vi "Begin.vi"(11 "Image Size":T1=enum."160x120") -> (0 "error out":errorcluster)   [LabVIEW 2012]
doc: "Called before other user functions, this VI is expected to open initial I/O refnums, load in file data, and do all program initialization. Notice that the <B>error out</B> terminal is simply used for data flow. Wiring it to other structures or subVIs ensures that this VI runs first."
uses:
  <vilib>/Rock Robotics/WPI/Camera/WPI_CameraImageSize.ctl
  <vilib>/Rock Robotics/WPI/Camera/WPI_CameraWhite Balance Values.ctl
  <vilib>/Rock Robotics/WPI/Camera/WPI_CameraExposure Values.ctl
  <vilib>/Rock Robotics/WPI/Camera/WPI_CameraFrameRate.ctl
  <vilib>/Rock Robotics/WPI/DriverStation/WPI_DriverStationRobotMode2.ctl
  <vilib>/Rock Robotics/WPI/Joystick/WPI_JoystickDeviceEnum.ctl
  <vilib>/Rock Robotics/SystemInterfaces/Typedef/FPGA_TypedefDigitalModule.ctl
  <vilib>/Rock Robotics/SystemInterfaces/DIO/FPGA_DIOPWMChannel.ctl
  <vilib>/Rock Robotics/WPI/Solenoid/WPI_SolenoidChannel.ctl
  <vilib>/Rock Robotics/SystemInterfaces/Typedef/FPGA_TypedefSolenoidModule.ctl
  <vilib>/Rock Robotics/SystemInterfaces/DIO/FPGA_DIOChannel.ctl
  <vilib>/Rock Robotics/WPI/Encoder/WPI_EncoderType.ctl
  <vilib>/Rock Robotics/WPI/SafetyOutput/WPI_SafetyOutputConfigMenu.ctl
  <vilib>/Rock Robotics/WPI/Solenoid/WPI_SolenoidValue.ctl
  <vilib>/Rock Robotics/SystemInterfaces/DIO/FPGA_DIORelayChannel.ctl
  <vilib>/Rock Robotics/SystemInterfaces/Typedef/FPGA_TypedefAnalogModuleForGyro.ctl
  <vilib>/Rock Robotics/SystemInterfaces/AI/FPGA_AIGyroChannel.ctl
  Robot Global Data.vi
  <vilib>/Rock Robotics/WPI/Solenoid/WPI_SolenoidOpenSingle.vi
  <vilib>/Rock Robotics/WPI/Solenoid/WPI_SolenoidSetEnum.vi
  <vilib>/Rock Robotics/WPI/Counter/WPI_CounterDigitalInputToDigitalSource.vi
  <vilib>/Rock Robotics/WPI/RobotDrive/WPI_RobotDriveOpen2MotorWithTalon.vi
  <vilib>/Rock Robotics/WPI/Solenoid/WPI_SolenoidOpenDouble.vi
  <vilib>/Rock Robotics/WPI/MotorControl/WPI_MotorControlOpen Talon.vi
  <vilib>/Rock Robotics/WPI/Compressor/WPI_CompressorGetSetRefNum.vi
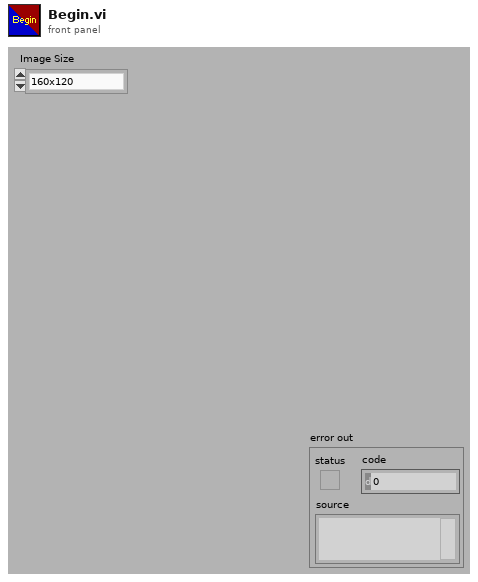
[diagram p1: front panel]
types:
  T1 = typedef "WPI_CameraImageSize.ctl" = enum16{"640x480", "320x240", "160x120"}
  T2 = typedef "WPI_SolenoidChannel.ctl" = enum8{"Solenoid 1", "Solenoid 2", "Solenoid 3", "Solenoid 4", "Solenoid 5", "Solenoid 6", "Solenoid 7", "Solenoid 8", "Invalid"}
  T3 = typedef "WPI_SolenoidValue.ctl" = enum16{"Off", "On", "Forward", "Reverse"}
  T4 = typedef "FPGA_AIGyroChannel.ctl" = enum8{"AI 1", "AI 2", "Invalid"}
  T5 = typedef "FPGA_TypedefAnalogModuleForGyro.ctl" = enum16{"Analog Module 1"}
  T6 = typedef "FPGA_DIOChannel.ctl" = enum8{"DIO 1", "DIO 2", "DIO 3", "DIO 4", "DIO 5", "DIO 6", "DIO 7", "DIO 8", "DIO 9", "DIO 10", "DIO 11", "DIO 12", "DIO 13", "DIO 14", "Invalid"}
  T7 = typedef "FPGA_DIORelayChannel.ctl" = enum8{"Relay 1", "Relay 2", "Relay 3", "Relay 4", "Relay 5", "Relay 6", "Relay 7", "Relay 8", "Invalid"}
  T8 = typedef "FPGA_TypedefDigitalModule.ctl" = enum16{"Digital Module 1", "Digital Module 2"}
  T9 = typedef "WPI_SafetyOutputConfigMenu.ctl" = enum16{"Enable", "Disable"}
  T10 = typedef "FPGA_DIOPWMChannel.ctl" = enum8{"PWM 1", "PWM 2", "PWM 3", "PWM 4", "PWM 5", "PWM 6", "PWM 7", "PWM 8", "PWM 9", "PWM 10", "Invalid"}
  T11 = typedef "WPI_EncoderType.ctl" = enum16{"1x", "2x", "4x"}
  T12 = typedef "FPGA_TypedefSolenoidModule.ctl" = enum16{"Solenoid Module 1", "Solenoid Module 2"}
  T13 = typedef "WPI_JoystickDeviceEnum.ctl" = enum16{"USB 1", "USB 2", "USB 3", "USB 4", "Kinect 1", "Kinect 2"}
  T14 = typedef "WPI_DriverStationRobotMode2.ctl" = enum16{"Autonomous Disabled", "Autonomous Enabled", "Teleop Disabled", "Teleop Enabled", "Timeout", "Finish", "Test Disabled", "Test Enabled"}
  T15 = typedef "WPI_CameraFrameRate.ctl" = u32
  T16 = typedef "WPI_CameraExposure Values.ctl" = enum16{"Auto", "Flicker-free 50 Hz", "Flicker-free 60 Hz", "Hold current"}
  T17 = typedef "WPI_CameraWhite Balance Values.ctl" = enum16{"Auto", "Fixed indoor", "Fixed outdoor 1", "Fixed outdoor 2", "Fixed fluorescent 1", "Fixed fluorescent 2", "Hold current"}
  T18 = typedef "WPI_DigitalInputDevRef.ctl" = cluster{"DevStatus":errorcluster, "DIO Channel":T6, "Digital Module":T8}
  T19 = typedef "WPI_CompressorDevRef.ctl" = cluster{"DevStatus":errorcluster, "DigitalInputDevRef":T18, "RelayDevRef":T20}
  T20 = typedef "WPI_RelayDevRef.ctl" = cluster{"DevStatus":errorcluster, "Relay Channel":T7, "Digital Module":T8, "Relay Direction":T21}
  T21 = typedef "WPI_RelayDirection.ctl" = enum16{"Both directions", "Forward only", "Reverse only"}
  T22 = typedef "FPGA_CounterEncoderSourceConvertionLVSourceType.ctl" = cluster{"DevStatus":errorcluster, "AnalogTriggerMode?":bool, "DigitalMode":cluster{"Digital Module":T8, "DIO Channel":T23}, "AnalogTriggerMode":cluster{"AnalogTriggerIndex":T24, "OutputType":T25}}
  T23 = typedef "FPGA_DIODigitalSourceChannel.ctl" = enum8{"DIO 1", "DIO 2", "DIO 3", "DIO 4", "DIO 5", "DIO 6", "DIO 7", "DIO 8", "DIO 9", "DIO 10", "DIO 11", "DIO 12", "DIO 13", "DIO 14", "Disabled"}
  T24 = typedef "FPGA_AnalogTriggerIndex.ctl" = enum8{"Trig 0", "Trig 1", "Trig 2", "Trig 3", "Trig 4", "Trig 5", "Trig 6", "Trig 7", "Invalid"}
  T25 = typedef "FPGA_AnalogTriggerOutType.ctl" = enum16{"InWindow", "TriggerState", "Rising", "Falling"}
  T26 = typedef "WPI_JoystickDevRef.ctl" = cluster{"Device":T13}
  T27 = typedef "WPI_CameraDevRef.ctl" = cluster{"Camera Address":string, "CameraStatus":errorcluster, "Acquire Image Notifier":refnum<notifier>}
  T28 = typedef "WPI_RobotDriveDevRef.ctl" = cluster{"DevStatus":errorcluster, "Motors[]":T29[], "Square Inputs":bool, "Max Output":dbl, "Isochronous":bool}
  T29 = typedef "WPI_MotorControlDeviceRef.ctl" = cluster{"DeviceStatus":errorcluster, "Type":enum16{"PWM", "CAN"}, "PWM":cluster{"Digital Module":T8, "PWM Channel":T10, "DeadBand":T30}, "CAN":cluster{"Device Number":u8, "Control Mode":T31, "Semaphore":T32, "Max Vout":dbl}, "Invert":bool, "TransformRef":T33, "InvTransformRef":T33}
  T30 = typedef "WPI_PWMDeadband.ctl" = cluster{"Name":string, "maxPositivePwm":i32, "minPositivePwm":i32, "centerPwm":i32, "maxNegativePwm":i32, "minNegativePwm":i32, "angularRange":u16}
  T31 = typedef "WPI_CANJaguar_ControlMode.ctl" = enum8{"Percent VBus", "Current", "Speed", "Position", "Voltage"}
  T32 = typedef "Semaphore RefNum" = refnum<k1>
  T33 = typedef "WPI_PWMTransform_ConPane.ctl" = refnum<vi>
  T34 = typedef "WPI_EncoderDevRef.ctl" = cluster{"DevStatus":errorcluster, "EncoderIndex":T35, "CounterIndex":T36, "DistancePerCount":dbl, "Decoding Type":T11}
  T35 = typedef "FPGA_EncoderIdx.ctl" = enum8{"Enc 0", "Enc 1", "Enc 2", "Enc 3", "Invalid"}
  T36 = typedef "FPGA_CounterCtrSystemIndex.ctl" = enum8{"Ctr 0", "Ctr 1", "Ctr 2", "Ctr 3", "Ctr 4", "Ctr 5", "Ctr 6", "Ctr 7", "Invalid"}
  T37 = typedef "WPI_SolenoidDevRef.ctl" = cluster{"DevStatus":errorcluster, "Solenoid Module":T12, "Forward Solenoid Channel":T2, "Reverse Solenoid Channel":T2}
  T38 = typedef "WPI_GyroDevRef.ctl" = cluster{"DevStatus":errorcluster, "Analog Module":T39, "Analog Channel":T40, "Offset":dbl, "Gain (VoltsPerDegree/Second)":dbl}
  T39 = typedef "FPGA_TypedefAnalogModule.ctl" = enum16{"Analog Module 1", "Analog Module 2"}
  T40 = typedef "FPGA_AIChannel.ctl" = enum8{"AI 1", "AI 2", "AI 3", "AI 4", "AI 5", "AI 6", "AI 7", "AI 8", "Invalid"}
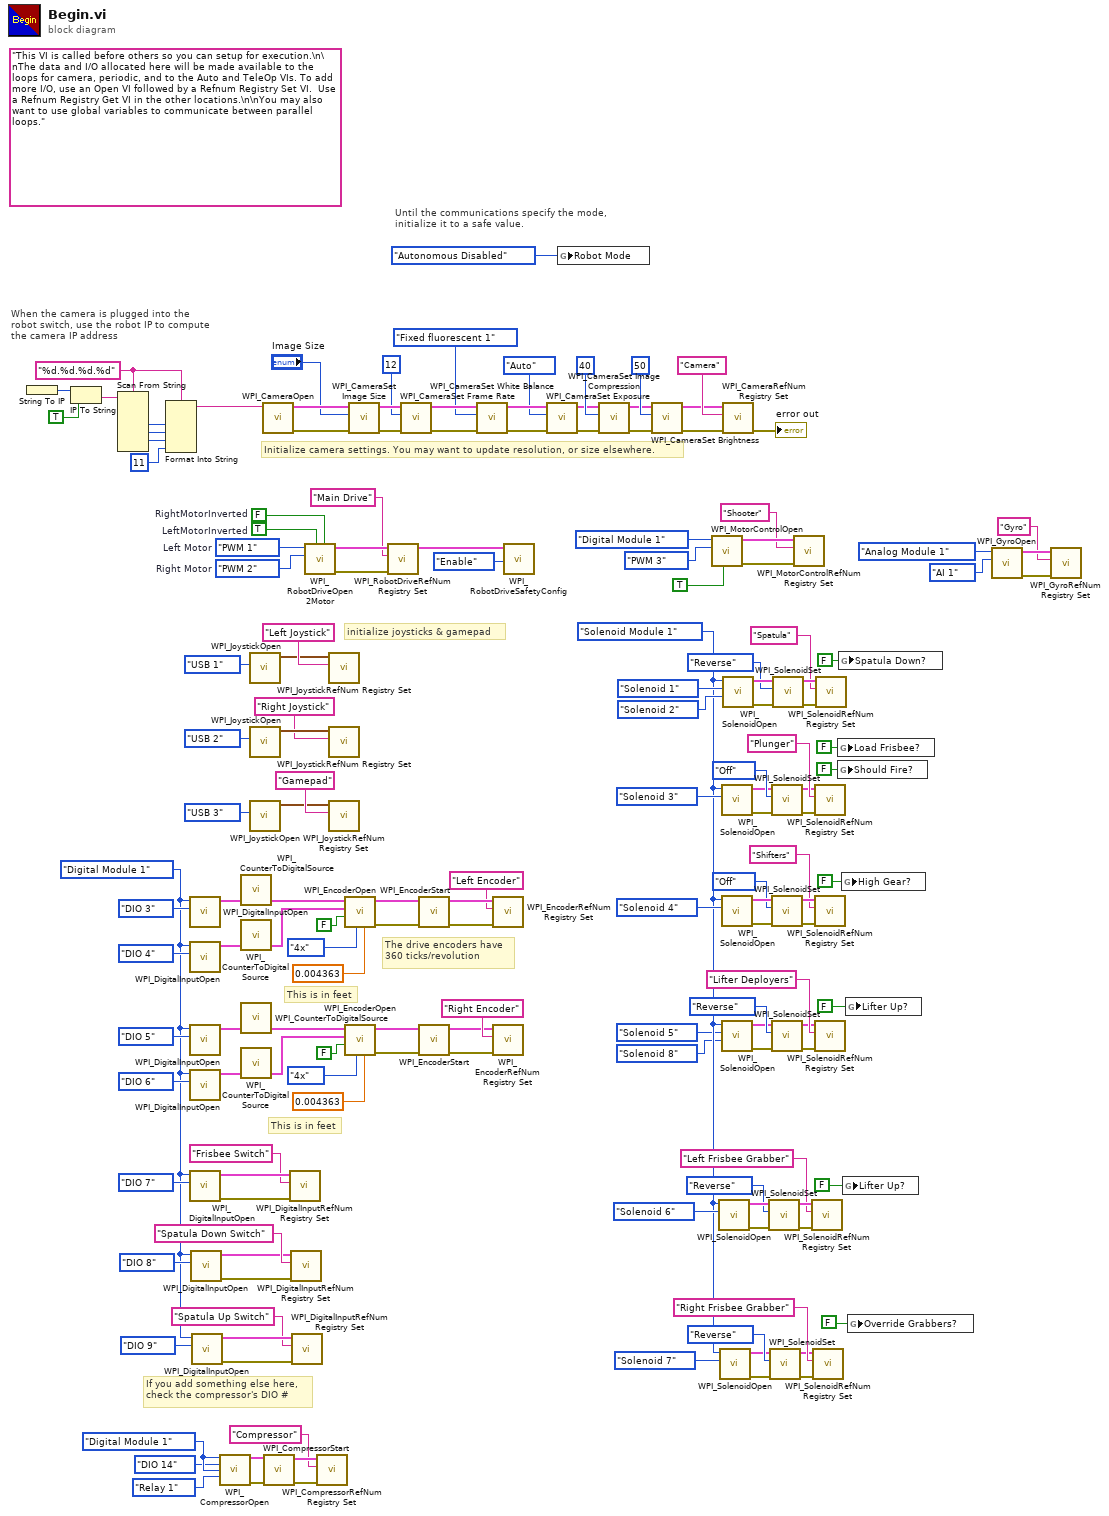
[diagram p0: block diagram]
diagram:
  w49 = FPGA_TypedefDigitalModule."Digital Module 1" ("Pressure Switch Digital Module (Module 1)")
  w67 = FPGA_DIOPWMChannel."PWM 2"  # Right Motor
  w68 = FPGA_DIOPWMChannel."PWM 1"  # Left Motor
  w72 = TRUE  # LeftMotorInverted
  w73 = FALSE  # RightMotorInverted
  w10 = FPGA_TypedefSolenoidModule."Solenoid Module 1" ("Solenoid Module (Module 1)")
  w33 = FPGA_TypedefDigitalModule."Digital Module 1" ("Digital Module (Module 1)")
  w134 = "%d.%d.%d.%d" ("format string")
  (unwired) "This VI is called before others so you can setup for execution.\n\nThe data and I/O allocated here will be made available to the loops for camera, periodic, and to the Auto and TeleOp VIs. To add more I/O, use an Open VI followed by a Refnum Registry Set VI.  Use a Refnum Registry Get VI in the other locations.\n\nYou may also want to use global variables to communicate between parallel loops."
  # "If you add something else here,\ncheck the compressor's DIO #"
  # "The drive encoders have\n360 ticks/revolution"
  # "This is in feet"
  # "This is in feet"
  # "initialize joysticks & gamepad"
  # "Until the communications specify the mode,\ninitialize it to a safe value."
  # "When the camera is plugged into the\nrobot switch, use the robot IP to compute\nthe camera IP address"
  # "Initialize camera settings. You may want to update resolution, or size elsewhere."
  n1 = String To IP() -> (0:w141:u32)  [unwired: 1 in]
  n2 = IP To String(1:TRUE ("dot notation? (F)"), 2:w141) -> (0:w139:string)
  n3 = Scan From String(format string=w134, input string=w139) -> (output 1=w138:i32, output 2=w137:i32, output 3=w136:i32)  [unwired: 7 in, 3 out]
  n4 = Format Into String(format string=w134, w138, w137, w136, 11 ("Compression")) -> (resulting string=w132:string)  [unwired: 2 in, 1 out]
  n5 = call <vilib>:"WPI_DigitalInputOpen.vi"("DIO Channel"=FPGA_DIOChannel."DIO 3" ("CS Channel"), "Digital Module (Module 1)"=w33) -> ("DigitalInputDevRef"=w95:T18)  [unwired: 1 in, 8 out]
  n6 = call <vilib>:"WPI_DigitalInputOpen.vi"("DIO Channel"=FPGA_DIOChannel."DIO 4" ("Clock Channel"), "Digital Module (Module 1)"=w33) -> ("DigitalInputDevRef"=w96:T18)  [unwired: 1 in, 8 out]
  n7 = call <vilib>:"WPI_DigitalInputOpen.vi"("DIO Channel"=FPGA_DIOChannel."DIO 5" ("CS Channel"), "Digital Module (Module 1)"=w33) -> ("DigitalInputDevRef"=w80:T18)  [unwired: 1 in, 8 out]
  n8 = call <vilib>:"WPI_DigitalInputOpen.vi"("DIO Channel"=FPGA_DIOChannel."DIO 6" ("Clock Channel"), "Digital Module (Module 1)"=w33) -> ("DigitalInputDevRef"=w79:T18)  [unwired: 1 in, 8 out]
  n9 = call <vilib>:"WPI_DigitalInputOpen.vi"("DIO Channel"=FPGA_DIOChannel."DIO 7", "Digital Module (Module 1)"=w33) -> ("error out"=w51:errorcluster, "DigitalInputDevRef"=w52:T18)  [unwired: 8 in]
  n10 = call <vilib>:"WPI_DigitalInputOpen.vi"("DIO Channel"=FPGA_DIOChannel."DIO 8", "Digital Module (Module 1)"=w33) -> ("error out"=w40:errorcluster, "DigitalInputDevRef"=w39:T18)  [unwired: 8 in]
  n11 = call <vilib>:"WPI_DigitalInputOpen.vi"("DIO Channel"=FPGA_DIOChannel."DIO 9", "Digital Module (Module 1)"=w33) -> ("error out"=w35:errorcluster, "DigitalInputDevRef"=w36:T18)  [unwired: 8 in]
  n12 = call <vilib>:"WPI_CompressorOpen.vi"("Pressure Switch Digital Module (Module 1)"=w49, "Pressure Switch DIO Channel"=FPGA_DIOChannel."DIO 14", "Relay Digital Module (Module 1)"=w49, "Relay Channel"=FPGA_DIORelayChannel."Relay 1") -> ("CompressorDevRef"=w45:T19, "error out"=w46:errorcluster)  [unwired: 10 in]
  n13 = call-poly <vilib>:"WPI_CounterToDigitalSource.vi"("DigitalInputDevRef"=w95) -> ("Digital Source"=w92:T22)  [unwired: 6 out]
  n14 = call-poly <vilib>:"WPI_CounterToDigitalSource.vi"("DigitalInputDevRef"=w96) -> ("Digital Source"=w93:T22)  [unwired: 6 out]
  n15 = call-poly <vilib>:"WPI_CounterToDigitalSource.vi"("DigitalInputDevRef"=w80) -> ("Digital Source"=w83:T22)  [unwired: 6 out]
  n16 = call-poly <vilib>:"WPI_CounterToDigitalSource.vi"("DigitalInputDevRef"=w79) -> ("Digital Source"=w82:T22)  [unwired: 6 out]
  n17 = call <vilib>:"WPI_JoystickOpen.vi"("JoystickDevice"=WPI_JoystickDeviceEnum."USB 1") -> ("JoystickDevRef"=w130:T26)  [unwired: 10 in]
  n18 = call <vilib>:"WPI_JoystickOpen.vi"("JoystickDevice"=WPI_JoystickDeviceEnum."USB 2") -> ("JoystickDevRef"=w126:T26)  [unwired: 10 in]
  n19 = call <vilib>:"WPI_JoystickOpen.vi"("JoystickDevice"=WPI_JoystickDeviceEnum."USB 3") -> ("JoystickDevRef"=w123:T26)  [unwired: 10 in]
  n20 = call <vilib>:"WPI_CameraOpen.vi"("Camera Address"=w132) -> ("error out"=w153:errorcluster, "CameraDevRef"=w154:T27)  [unwired: 1 in, 8 out]
  n21 = call <vilib>:"WPI_CompressorStart.vi"("error in (no error)"=w46, "CompressorDevRef"=w45) -> ("error out"=w44:errorcluster, "CompressorDevRef"=w43:T19)  [unwired: 8 in]
  n22 = call <vilib>:"WPI_DigitalInputRefNum Registry Set.vi"("error in (no error)"=w51, "refnum name"="Frisbee Switch", "DigitalInputDevRef"=w52) -> ()  [unwired: 7 in, 2 out]
  n23 = call <vilib>:"WPI_DigitalInputRefNum Registry Set.vi"("error in (no error)"=w40, "refnum name"="Spatula Down Switch", "DigitalInputDevRef"=w39) -> ()  [unwired: 7 in, 2 out]
  n24 = call <vilib>:"WPI_DigitalInputRefNum Registry Set.vi"("error in (no error)"=w35, "refnum name"="Spatula Up Switch", "DigitalInputDevRef"=w36) -> ()  [unwired: 7 in, 2 out]
  n25 = call-poly <vilib>:"WPI_RobotDriveOpen2Motor.vi"("Right Motor Inverted"=w73, "Left Motor Inverted"=w72, "Right Motor"=w67, "Left Motor"=w68) -> ("error out"=w69:errorcluster, "RobotDriveDevRef"=w71:T28)  [unwired: 1 in, 5 out]
  n26 = call <vilib>:"WPI_CompressorRefNum Registry Set.vi"("error in (no error)"=w44, "refnum name"="Compressor", "CompressorDevRef"=w43) -> ()  [unwired: 7 in, 2 out]
  n27 = call <vilib>:"WPI_JoystickRefNum Registry Set.vi"("refnum name"="Left Joystick", "JoystickDevRef"=w130) -> ()  [unwired: 8 in, 2 out]
  n28 = call <vilib>:"WPI_JoystickRefNum Registry Set.vi"("refnum name"="Right Joystick", "JoystickDevRef"=w126) -> ()  [unwired: 8 in, 2 out]
  n29 = call <vilib>:"WPI_JoystickRefNum Registry Set.vi"("refnum name"="Gamepad", "JoystickDevRef"=w123) -> ()  [unwired: 8 in, 2 out]
  n30 = call <vilib>:"WPI_EncoderOpen.vi"("DistancePerCount"=0.004363, "Decoding Type"=WPI_EncoderType."4x", "Invert Direction (False)"=FALSE, "BSource"=w93, "ASource"=w92) -> ("error out"=w98:errorcluster, "EncoderDevRef"=w97:T34)  [unwired: 5 in]
  n31 = call <vilib>:"WPI_EncoderOpen.vi"("DistancePerCount"=0.004363, "Decoding Type"=WPI_EncoderType."4x", "Invert Direction (False)"=FALSE, "BSource"=w82, "ASource"=w83) -> ("error out"=w77:errorcluster, "EncoderDevRef"=w78:T34)  [unwired: 5 in]
  n32 = call <vilib>:"WPI_CameraSet Image Size.vi"("error in (no error)"=w153, "Image Size"="Image Size", "CameraDevRef"=w154) -> ("error out"=w152:errorcluster, "CameraDevRef Out"=w155:T27)  [unwired: 7 out]
  n33 = call <vilib>:"WPI_RobotDriveRefNum Registry Set.vi"("error in (no error)"=w69, "refnum name"="Main Drive", "RobotDriveDevRef"=w71) -> ("RobotDriveDevRef"=w66:T28)  [unwired: 8 out]
  n34 = call <vilib>:"WPI_CameraSet Frame Rate.vi"("error in (no error)"=w152, "Frame Rate (fps)"=T15 12, "CameraDevRef"=w155) -> ("error out"=w151:errorcluster, "CameraDevRef Out"=w157:T27)  [unwired: 7 out]
  n35 = call <vilib>:"WPI_EncoderStart.vi"("error in (no error)"=w98, "EncoderDevRef"=w97) -> ("error out"=w99:errorcluster, "EncoderDevRef"=w100:T34)  [unwired: 8 in]
  n36 = call <vilib>:"WPI_EncoderStart.vi"("error in (no error)"=w77, "EncoderDevRef"=w78) -> ("error out"=w76:errorcluster, "EncoderDevRef"=w75:T34)  [unwired: 8 in]
  n37 = call <vilib>:"WPI_CameraSet White Balance.vi"("error in (no error)"=w151, "White Balance"=WPI_CameraWhite_Balance_Values."Fixed fluorescent 1", "CameraDevRef"=w157) -> ("error out"=w150:errorcluster, "CameraDevRef Out"=w156:T27)  [unwired: 7 out]
  n38 = call <vilib>:"WPI_EncoderRefNum Registry Set.vi"("error in (no error)"=w99, "refnum name"="Left Encoder", "EncoderDevRef"=w100) -> ()  [unwired: 7 in, 2 out]
  n39 = call <vilib>:"WPI_EncoderRefNum Registry Set.vi"("error in (no error)"=w76, "refnum name"="Right Encoder", "EncoderDevRef"=w75) -> ()  [unwired: 7 in, 2 out]
  n40 = call <vilib>:"WPI_RobotDriveSafetyConfig.vi"("mode"=WPI_SafetyOutputConfigMenu."Enable", "RobotDriveDevRef"=w66) -> ()  [unwired: 8 in, 2 out]
  n41 = call <vilib>:"WPI_CameraSet Exposure.vi"("error in (no error)"=w150, "Exposure"=WPI_CameraExposure_Values."Auto", "CameraDevRef"=w156) -> ("error out"=w149:errorcluster, "CameraDevRef Out"=w159:T27)  [unwired: 7 out]
  n42 = global write "Robot Global Data.vi" "Robot Mode"(WPI_DriverStationRobotMode2."Autonomous Disabled" ("Robot Mode")) -> ()
  n43 = call <vilib>:"WPI_CameraSet Image Compression.vi"("error in (no error)"=w149, "Compression"=40, "CameraDevRef"=w159) -> ("error out"=w148:errorcluster, "CameraDevRef Out"=w158:T27)  [unwired: 7 out]
  n44 = call <vilib>:"WPI_CameraSet Brightness.vi"("error in (no error)"=w148, "Brightness"=50, "CameraDevRef"=w158) -> ("error out"=w146:errorcluster, "CameraDevRef Out"=w147:T27)  [unwired: 7 out]
  n45 = call-poly <vilib>:"WPI_MotorControlOpen.vi"("Invert"=TRUE, "PWM Channel"=FPGA_DIOPWMChannel."PWM 3", "Digital Module (Module 1)"=FPGA_TypedefDigitalModule."Digital Module 1") -> ("error out"=w118:errorcluster, "MotorControlDeviceRef"=w119:T29)  [unwired: 7 in]
  n46 = call-poly <vilib>:"WPI_SolenoidOpen.vi"("Solenoid Channel"=WPI_SolenoidChannel."Solenoid 6", "Solenoid Module (Module 1)"=w10) -> ("error out"=w23:errorcluster, "SolenoidDevRef"=w24:T37)  [unwired: 8 in]
  n47 = call-poly <vilib>:"WPI_SolenoidOpen.vi"("Solenoid Channel"=WPI_SolenoidChannel."Solenoid 7", "Solenoid Module (Module 1)"=w10) -> ("error out"=w14:errorcluster, "SolenoidDevRef"=w13:T37)  [unwired: 8 in]
  n48 = call-poly <vilib>:"WPI_SolenoidOpen.vi"("Solenoid Channel"=WPI_SolenoidChannel."Solenoid 3", "Solenoid Module (Module 1)"=w10) -> ("error out"=w106:errorcluster, "SolenoidDevRef"=w105:T37)  [unwired: 8 in]
  n49 = call-poly <vilib>:"WPI_SolenoidOpen.vi"("Solenoid Channel"=WPI_SolenoidChannel."Solenoid 4", "Solenoid Module (Module 1)"=w10) -> ("error out"=w61:errorcluster, "SolenoidDevRef"=w62:T37)  [unwired: 8 in]
  n50 = call-poly <vilib>:"WPI_SolenoidOpen.vi"("Reverse Solenoid Channel"=WPI_SolenoidChannel."Solenoid 8", "Forward Solenoid Channel"=WPI_SolenoidChannel."Solenoid 5" ("Solenoid Channel"), "Solenoid Module (Module 1)"=w10) -> ("error out"=w5:errorcluster, "SolenoidDevRef"=w4:T37)  [unwired: 7 in]
  n51 = call <vilib>:"WPI_CameraRefNum Registry Set.vi"("error in (no error)"=w146, "refnum name"="Camera", "CameraDevRef"=w147) -> ("error out"=→"error out":errorcluster)  [unwired: 8 out]
  n52 = call-poly <vilib>:"WPI_SolenoidOpen.vi"("Reverse Solenoid Channel"=WPI_SolenoidChannel."Solenoid 2", "Forward Solenoid Channel"=WPI_SolenoidChannel."Solenoid 1" ("Solenoid Channel"), "Solenoid Module (Module 1)"=w10) -> ("error out"=w114:errorcluster, "SolenoidDevRef"=w115:T37)  [unwired: 7 in]
  n53 = call-poly <vilib>:"WPI_SolenoidSet.vi"("error in (no error)"=w23, "Value"=WPI_SolenoidValue."Reverse", "SolenoidDevRef"=w24) -> ("error out"=w22:errorcluster, "SolenoidDevRef"=w21:T37)  [unwired: 7 in]
  n54 = call-poly <vilib>:"WPI_SolenoidSet.vi"("error in (no error)"=w14, "Value"=WPI_SolenoidValue."Reverse", "SolenoidDevRef"=w13) -> ("error out"=w15:errorcluster, "SolenoidDevRef"=w16:T37)  [unwired: 7 in]
  n55 = call-poly <vilib>:"WPI_SolenoidSet.vi"("error in (no error)"=w106, "Value"=WPI_SolenoidValue."Off", "SolenoidDevRef"=w105) -> ("error out"=w107:errorcluster, "SolenoidDevRef"=w108:T37)  [unwired: 7 in]
  n56 = call-poly <vilib>:"WPI_SolenoidSet.vi"("error in (no error)"=w61, "Value"=WPI_SolenoidValue."Off", "SolenoidDevRef"=w62) -> ("error out"=w60:errorcluster, "SolenoidDevRef"=w59:T37)  [unwired: 7 in]
  n57 = call-poly <vilib>:"WPI_SolenoidSet.vi"("error in (no error)"=w5, "Value"=WPI_SolenoidValue."Reverse", "SolenoidDevRef"=w4) -> ("error out"=w6:errorcluster, "SolenoidDevRef"=w7:T37)  [unwired: 7 in]
  n58 = call-poly <vilib>:"WPI_SolenoidSet.vi"("error in (no error)"=w114, "Value"=WPI_SolenoidValue."Reverse", "SolenoidDevRef"=w115) -> ("error out"=w113:errorcluster, "SolenoidDevRef"=w112:T37)  [unwired: 7 in]
  n59 = call <vilib>:"WPI_MotorControlRefNum Registry Set.vi"("error in (no error)"=w118, "refnum name"="Shooter", "MotorControlDevRef"=w119) -> ()  [unwired: 7 in, 2 out]
  n60 = call <vilib>:"WPI_SolenoidRefNum Registry Set.vi"("error in (no error)"=w22, "refnum name"="Left Frisbee Grabber", "SolenoidDevRef"=w21) -> ()  [unwired: 7 in, 2 out]
  n61 = call <vilib>:"WPI_SolenoidRefNum Registry Set.vi"("error in (no error)"=w15, "refnum name"="Right Frisbee Grabber", "SolenoidDevRef"=w16) -> ()  [unwired: 7 in, 2 out]
  n62 = call <vilib>:"WPI_SolenoidRefNum Registry Set.vi"("error in (no error)"=w107, "refnum name"="Plunger", "SolenoidDevRef"=w108) -> ()  [unwired: 7 in, 2 out]
  n63 = call <vilib>:"WPI_SolenoidRefNum Registry Set.vi"("error in (no error)"=w60, "refnum name"="Shifters", "SolenoidDevRef"=w59) -> ()  [unwired: 7 in, 2 out]
  n64 = call <vilib>:"WPI_SolenoidRefNum Registry Set.vi"("error in (no error)"=w6, "refnum name"="Lifter Deployers", "SolenoidDevRef"=w7) -> ()  [unwired: 7 in, 2 out]
  n65 = call <vilib>:"WPI_SolenoidRefNum Registry Set.vi"("error in (no error)"=w113, "refnum name"="Spatula", "SolenoidDevRef"=w112) -> ()  [unwired: 7 in, 2 out]
  n66 = global write "Robot Global Data.vi" "Load Frisbee?"(FALSE ("High Gear?")) -> ()
  n67 = global write "Robot Global Data.vi" "Should Fire?"(FALSE ("High Gear?")) -> ()
  n68 = global write "Robot Global Data.vi" "Spatula Down?"(FALSE ("High Gear?")) -> ()
  n69 = global write "Robot Global Data.vi" "High Gear?"(FALSE ("High Gear?")) -> ()
  n70 = global write "Robot Global Data.vi" "Lifter Up?"(FALSE ("High Gear?")) -> ()
  n71 = global write "Robot Global Data.vi" "Lifter Up?"(FALSE ("High Gear?")) -> ()
  n72 = global write "Robot Global Data.vi" "Override Grabbers?"(FALSE ("High Gear?")) -> ()
  n73 = call <vilib>:"WPI_GyroOpen.vi"("Analog Channel"=FPGA_AIGyroChannel."AI 1", "Analog Module (Module 1)"=FPGA_TypedefAnalogModuleForGyro."Analog Module 1") -> ("error out"=w31:errorcluster, "GyroDevRef"=w30:T38)  [unwired: 7 in, 1 out]
  n74 = call <vilib>:"WPI_GyroRefNum Registry Set.vi"("error in (no error)"=w31, "refnum name"="Gyro", "GyroDevRef"=w30) -> ()  [unwired: 7 in, 2 out]
